vi "my_highpass.vi"(7 "input":dbl format="%.2f", 13 "corner period (steps)":dbl(slide)=10.237739663395852 scale=1.0..1000.0) -> (8 "output":dbl format="%.2f")   [LabVIEW 2017]
doc: "This is a high pass filter using ITR first order derivation."
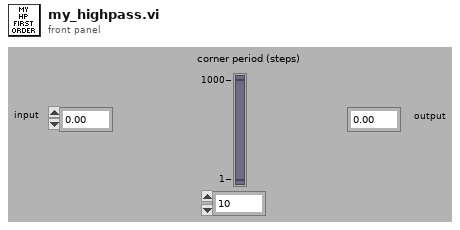
[diagram p1: front panel]
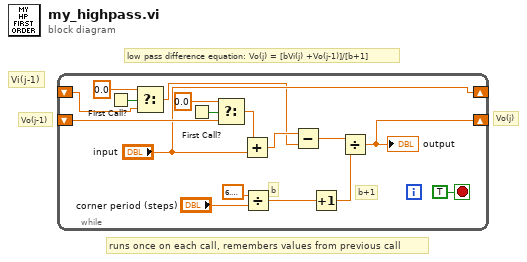
[diagram p0: block diagram]
diagram:
  # "Vi(j-1)"
  # "runs once on each call, remembers values from previous call"
  # "Vo(j-1)"
  # "Vo(j)"
  # "low pass difference equation: Vo(j) = [bVi(j) +Vo(j-1)]/[b+1]"
  n1 = while {
    shift-left: _ -> [w10]
    shift-right: [w12] -> _
    shift-right: ["input"] -> _
    shift-left: _ -> [w5]
    stop <- TRUE stop-if-true
    # "b+1"
    # "b"
    n2 = First Call?() -> (First Call?: T/F=w6:bool)
    n3 = Select(t=0.0, s=w6, f=w5) -> (s? t:f=w1:dbl)
    n4 = First Call?() -> (First Call?: T/F=w11:bool)
    n5 = Select(t=0.0, s=w11, f=w10) -> (s? t:f=w9:dbl)
    n6 = Add(x=w9, y="input") -> (x+y=w2:dbl)
    n7 = Divide(x=6.283185307179586, y="corner period (steps)") -> (x/y=w14:dbl)
    n8 = Subtract(x=w2, y=w1) -> (x-y=w3:dbl)
    n9 = Increment(x=w14) -> (x+1=w13:dbl)
    n10 = Divide(x=w3, y=w13) -> (x/y=w12:dbl)
    "output" <- w12
  }
